vi "Initialize Text File.vi"(7 "operation (0:open)":T1(ring), 8 "error in (no error)":errorcluster, 10 "file path (use dialog)":path, 11 "Text File in":refnum<class "Text File.lvclass">) -> (0 "error out":errorcluster, 3 "Text File out":refnum<class "Text File.lvclass">)   [LabVIEW 2020, in "Text File.lvclass"]
uses:
  <vilib>/gpm_packages/@cs/event-logger/Source/Text File Sink/Text File/Text File.lvclass
  <vilib>/gpm_packages/@cs/event-logger/Source/Text File Sink/Text File/Text File.lvclass/Text File.ctl
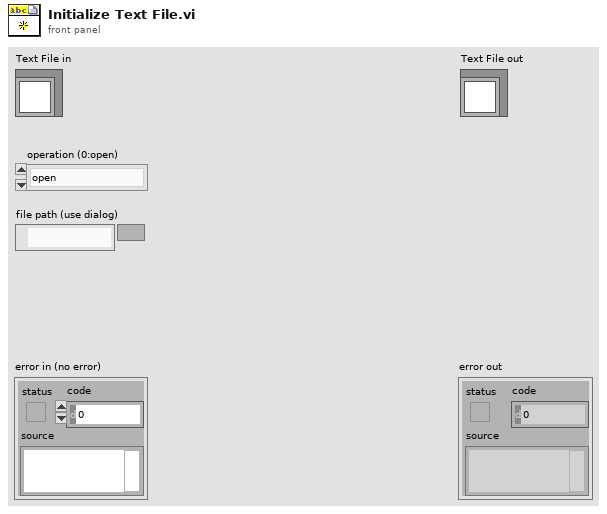
[diagram p1: front panel]
types:
  T1 = enum16{"open", "replace", "create", "open or create", "replace or create", "replace or create with confirmation"}
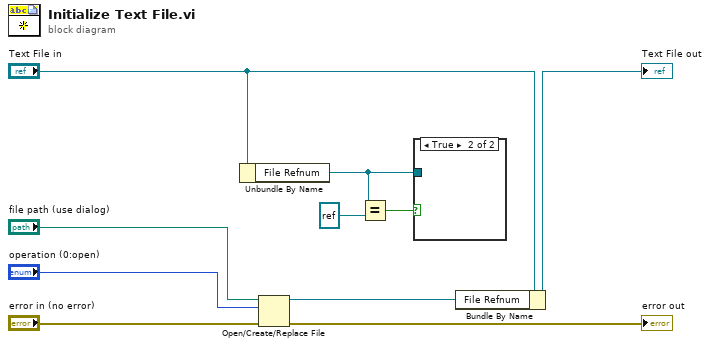
[diagram p0: block diagram]
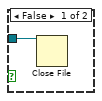
[diagram p2: hidden frame]
diagram:
  n1 = Unbundle By Name("Text File in") -> ("File Refnum"=w1:refnum<file>)
  n2 = Open/Create/Replace File(file path (use dialog)="file path (use dialog)", error in="error in (no error)", operation (0:open)="operation (0:open)") -> (refnum out=w5:refnum<file>, error out=→"error out":errorcluster)  [unwired: 3 in, 1 out]
  n3 = Equal?(x=w1, y=refnum<file> refnum) -> (x = y?=w2:bool)
  n4 = case shown="True" w2 {
    tunnel: w1 -> [w11 _]
    frame False {
      n5 = Close File(refnum=w11) -> ()  [unwired: 1 in, 2 out]
    }
    frame True {
    }
  }
  n6 = Bundle By Name(cluster="Text File in", "File Refnum"=w5) -> (→"Text File out":refnum<class "Text File.lvclass">)
